vi "PlaceChar.vi"(9 "cursor in":i32, 10 "value":u8, 11 "Array in":u8[](array[numeric])) -> (3 "Array out":u8[](array[numeric]))   [LabVIEW 2021]
panel:
  out "String Out":string
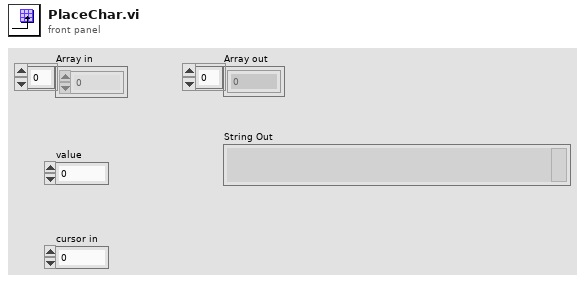
[diagram p1: front panel]
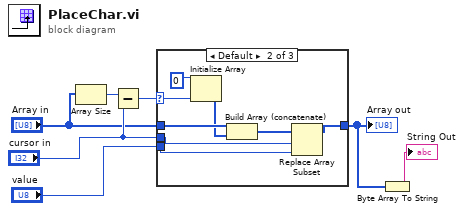
[diagram p0: block diagram]
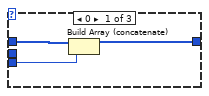
[diagram p2: hidden frame]
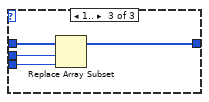
[diagram p3: hidden frame]
diagram:
  n1 = Array Size(array="Array in") -> (size(s)=w5:i32)
  n2 = Subtract(x=w5, y="cursor in") -> (x-y=w7:i32)
  n3 = case shown="Default" w7 {
    selector: w7 -> [_ w18 _]
    tunnel: "value" -> [w9 w11 w22]
    tunnel: [w8 w13 w21] -> w1
    tunnel: "Array in" -> [w10 w17 w20]
    tunnel: "cursor in" -> [_ w12 w19]
    frame 0 {
      n4 = Build Array (concatenate)(w10, w9) -> (w8:u8[])
    }
    frame Default {
      n5 = Initialize Array(u8 0, w18) -> (w16:u8[])
      n6 = Build Array (concatenate)(w17, w16) -> (w14:u8[])
      n7 = Replace Array Subset(array=w14, new element=w11, index=w12) -> (w13:u8[])
    }
    frame 1.. {
      n8 = Replace Array Subset(array=w20, new element=w22, index=w19) -> (w21:u8[])
    }
  }
  "Array out" <- w1
  n9 = Byte Array To String(unsigned byte array=w1) -> (string=→"String Out":string)
